vi "ThresholdAviMesure.vi"() -> ()   [LabVIEW 2015]
uses:
  <vilib>/vision/NI_Vision_Development_Module.lvlib
  <vilib>/ptbypt/NI_PtbyPt.lvlib
panel:
  out "Numero de Macthes 2":i32
  out "Dif. CM":dbl
  in  "x":i32=20
  out "Dif. Puntos":i32
  out "2°":i32
  out "1°":i32
  out "Global Rectangle":dbl[](array[numeric])
  in  "Tab Control":T1(tab)
  out "Waveform Chart":dbl(graph)
  out "Waveform Chart 2":dbl(graph)
  out "Waveform Chart 3":dbl(graph)
  out "Waveform Graph":dbl[](graph)
  out "Saving Data":bool
  in  "Filename":path=path "C:/Users/denni/Google Drive/ProyectoEspi/Dennis/Espirometro.lvm/Medidas.xlsx"
  out "Dist. CM":sgl
  out "Dist. Pixel":sgl
  out "Image 2":T2(plugin-control)
  out "Image":T2(plugin-control)
  out "Barra de Progreso":i32(slide) max=1548 scale=-1.0..1548.0
  out "SNAP 1":bool
  out "SNAP 2":bool
  out "Numero de Macthes":i32
  out "Coordenadas":T3(array[cluster]) {"Position"."Y" format="%.2f"; "Position"."X" format="%.2f"}
  in  "REC":bool=TRUE
  in  "SNAP 1":bool=TRUE
  in  "Stop Button":bool
  in  "Minimum Score":sgl=700.0
  in  "Max # of Matches":i32=1
  out "Threshold":T2(plugin-control)
  out "Original":T2(plugin-control)
  in  "Blue or Luminance":cluster{i32, i32}(slide)={30, 255} scale=0.0..255.0
  in  "Green or Saturation":cluster{i32, i32}(slide)={100, 255} scale=0.0..255.0
  in  "Threshold Color Mode":enum32{"RGB", "HSL"}(radio)=enum."HSL"
  in  "Red or Hue":cluster{i32, i32}(slide)={90, 222} scale=0.0..255.0
  out "error out":errorcluster
  in  "error in (no error)":errorcluster
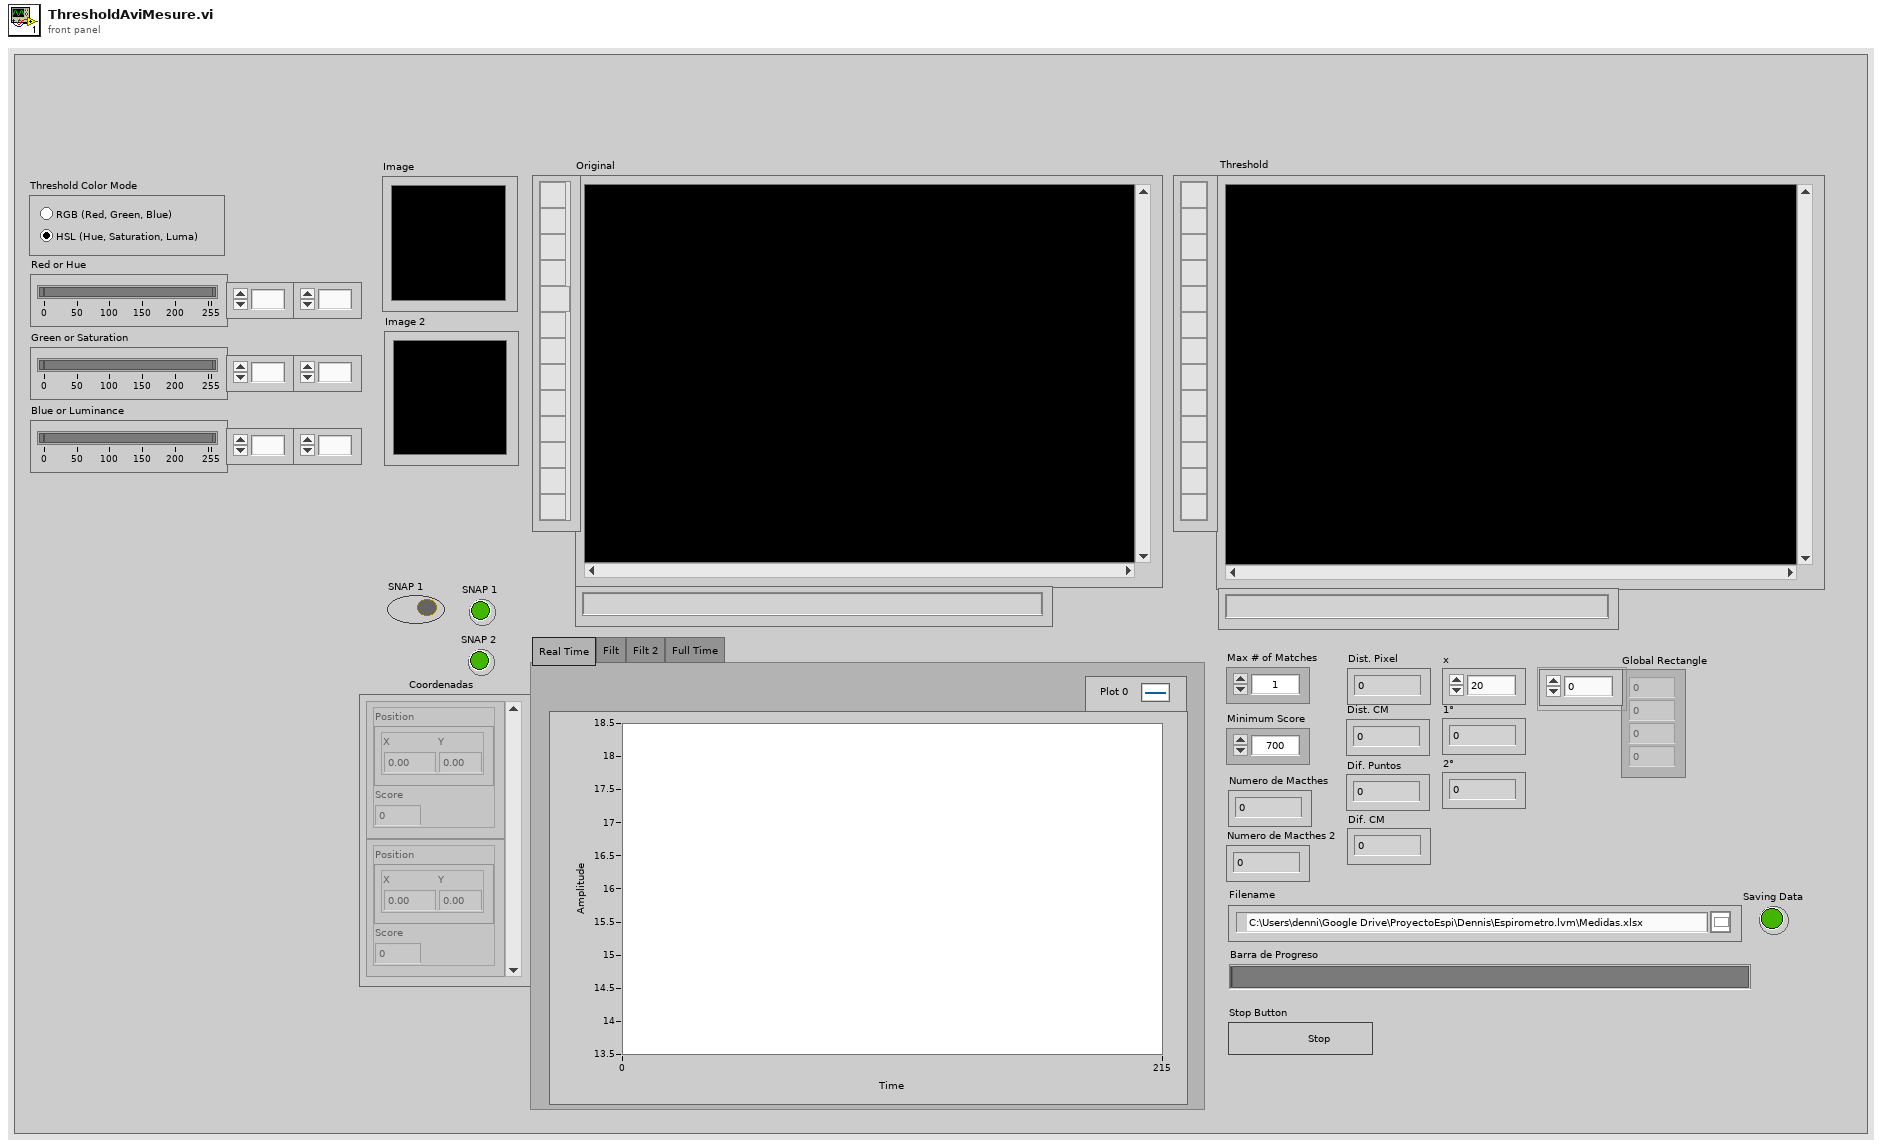
[diagram p1: front panel]
types:
  T1 = enum32{"Real Time", "Filt", "Filt 2", "Full Time"}
  T2 = typedef "IMAQ Image.ctl" = refnum<image>
  T3 = cluster{"Position":cluster{"X":dbl, "Y":dbl}, "Score":dbl}[]
  T4 = typedef "Image Type" = u32
  T5 = typedef "IMAQ AVI2 Refnum.ctl" = refnum<k20>
  T6 = cluster{"Global Rectangle":i32[], "Contours":cluster{"Contour Type":u32, "ROI Type":u32, "Points":i32[]}[]}
  T7 = cluster{"Position":cluster{"x":sgl, "y":sgl}, "Angle":sgl, "Scale":sgl, "Score":sgl, "Bounding Box":cluster{"x":sgl, "y":sgl}[]}[]
  T8 = cluster{"Position":cluster{"x":sgl, "y":sgl}, "Angle":sgl}
  T9 = cluster{"Position":cluster{"x":sgl, "y":sgl}, "Angle":sgl, "Scale":sgl, "Score":sgl, "Bounding Box":cluster{"x":sgl, "y":sgl}[]}
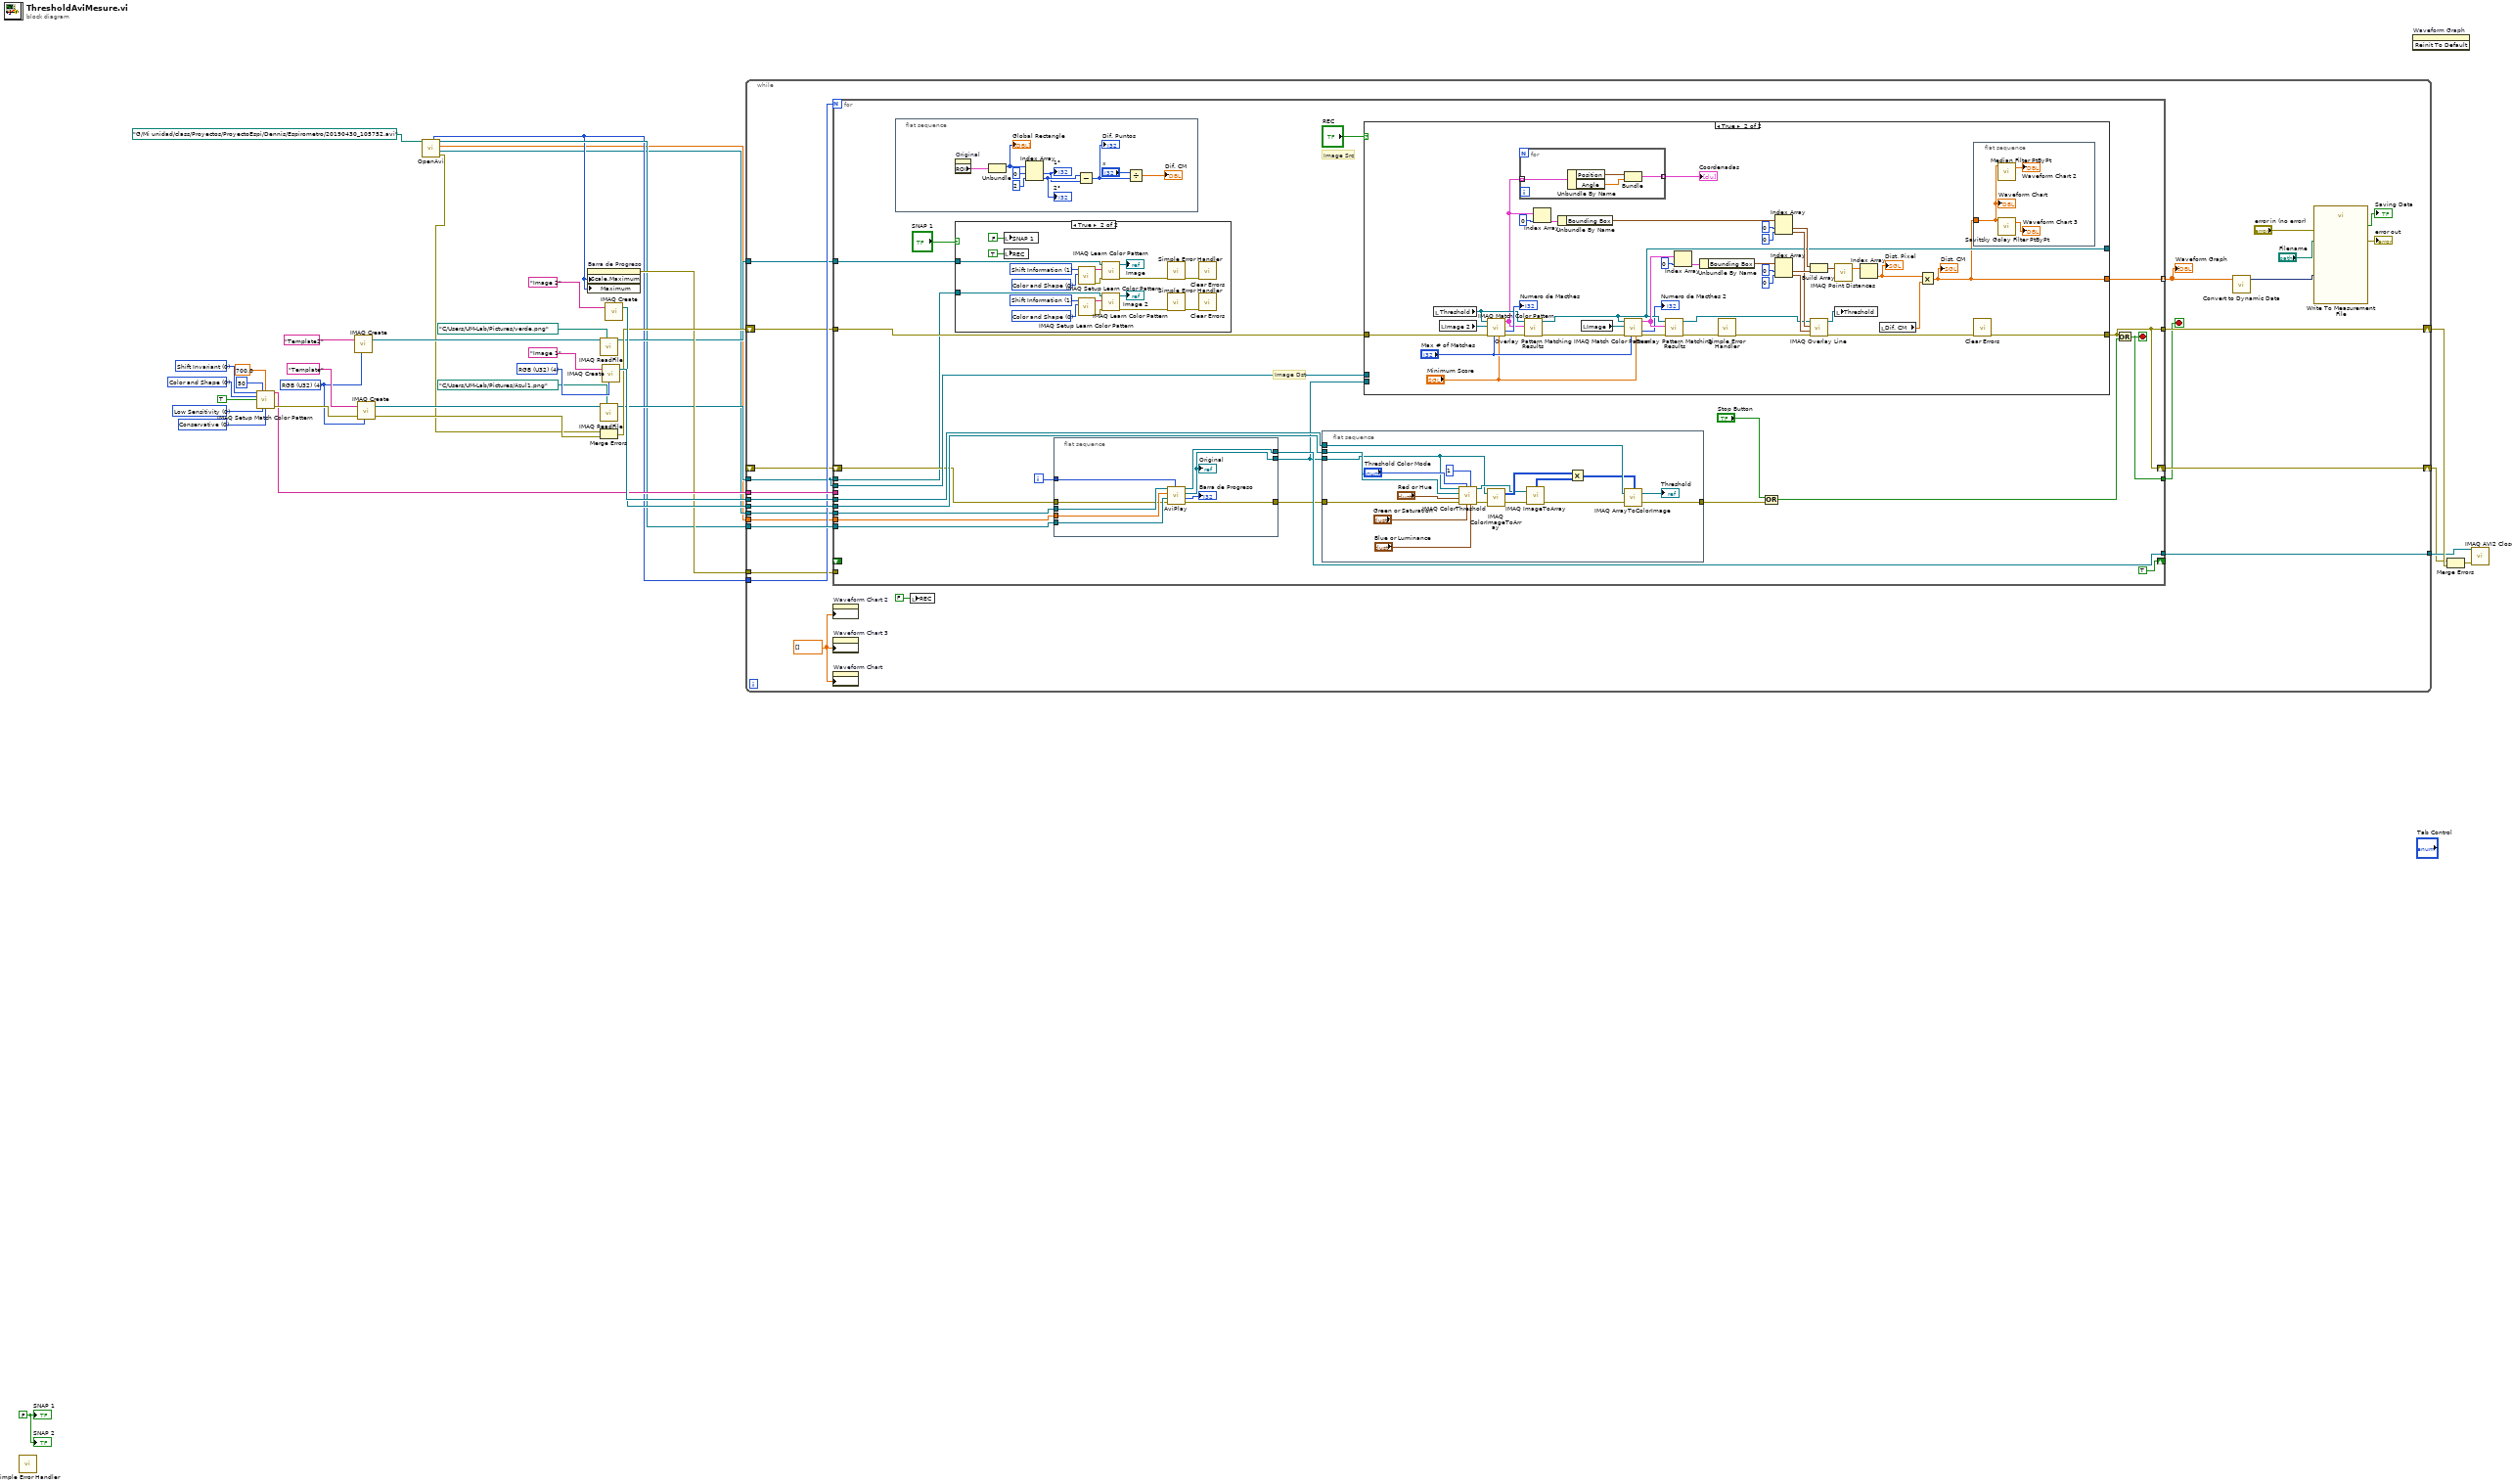
[diagram p0: block diagram]
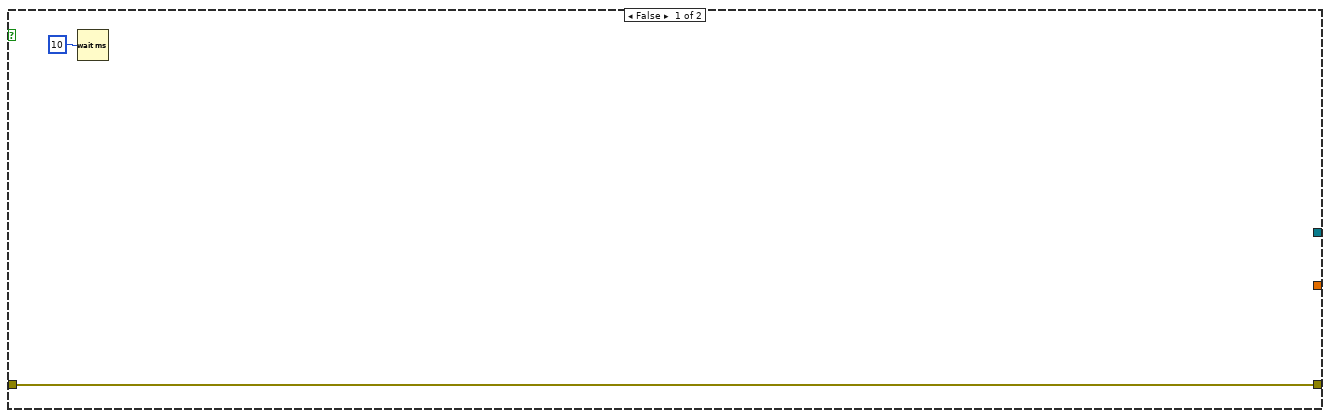
[diagram p3: hidden frame]
diagram:
  w17 = FALSE
  w24 = u32 0 items=["Shift Invariant", "Rotation Invariant"] ("Match Mode")
  w26 = u32 0 items=["Color and Shape", "Color", "Shape"] ("Match Feature Mode")
  w27 = u32 0 items=["Conservative", "Balance", "Aggressive", "Very Aggressive"] ("Search Strategy")
  w28 = u32 0 items=["Low Sensitivity", "Medium Sensitivity", "High Sensitivity"] ("Color Sensitivity")
  w18 = T4 4 items=["Grayscale (U8)", "Grayscale (I16)", "Grayscale (SGL)", "Complex (CSG)", "RGB (U32)", "HSL (U32)", "RGB (U64)", "Grayscale (U16)"] ("Image Type")
  w36 = T4 4 items=["Grayscale (U8)", "Grayscale (I16)", "Grayscale (SGL)", "Complex (CSG)", "RGB (U32)", "HSL (U32)", "RGB (U64)", "Grayscale (U16)"] ("Image Type")
  n1 = call <vilib>:"Simple Error Handler.vi"() -> ()  [unwired: 5 in, 5 out]
  n2 = call "IMAQ Setup Match Color Pattern"("Match Mode"=w24, "Minimum Contrast"=50, "Color Score Weight"=sgl 700.0, "Match Feature Mode"=w26, "Subpixel Accuracy"=TRUE, "Color Sensitivity"=w28, "Search Strategy"=w27) -> ("Match Color Pattern Setup Data"=w29:string, "error out"=w31:errorcluster)  [unwired: 7 in]
  n3 = call "IMAQ Create"("Image Name"="Template2", "Image Type"=w18) -> ("New Image"=w11:T2)  [unwired: 3 in, 1 out]
  n4 = call "IMAQ Create"("Image Name"="Template", "Image Type"=w18, "error in (no error)"=w31) -> ("New Image"=w13:T2, "error out"=w30:errorcluster)  [unwired: 2 in]
  n5 = call "OpenAvi.vi"("Example Image Path"=path "G:/Mi unidad/class/Proyectos/ProyectoEspi/Dennis/Espirometro/20190430_105752.avi" ("base path")) -> ("error out"=w5:errorcluster, "AVI Refnum (duplicate)"=w3:T5, "Sec per Frame"=w2:dbl, "Refnum out Image"=w6:T2, "Number of Frames For"=w4:u32)  [unwired: 6 in]
  n6 = property on="Barra de Progreso" class="Slide (strict)"("Scale.Maximum"=w4, "Maximum"=w4) -> (error out=w16:errorcluster)  [unwired: 2 in, 1 out]
  n7 = call "IMAQ ReadFile"("File Path"=path "C:/Users/UM-Lab/Pictures/verde.png", "Image"=w11) -> ("Image Out"=w10:T2)  [unwired: 5 in, 4 out]
  n8 = call "IMAQ ReadFile"("File Path"=path "C:/Users/UM-Lab/Pictures/Azul1.png", "Image"=w13) -> ("Image Out"=w12:T2)  [unwired: 5 in, 4 out]
  n9 = Merge Errors(w5, w30) -> (w21:errorcluster)
  n10 = call "IMAQ Create"("Image Name"="Image 1", "Image Type"=w36) -> ("New Image"=w35:T2)  [unwired: 3 in, 1 out]
  n11 = call "IMAQ Create"("Image Name"="Image 2") -> ("New Image"=w33:T2)  [unwired: 4 in, 1 out]
  n12 = while {
    tunnel: w35 -> [w61]
    tunnel: w33 -> [w60]
    tunnel: w29 -> [w59]
    tunnel: w12 -> [w42]
    tunnel: w10 -> [w41]
    tunnel: w6 -> [w56]
    tunnel: w4 -> [w55]
    tunnel: w16 -> [w54]
    tunnel: w2 -> [w53]
    tunnel: w3 -> [w52]
    shift-right: [w58] -> w20
    shift-left: w21 -> [w43]
    shift-right: [w57] -> w1
    shift-left: _ -> [w51]
    tunnel: [w50] -> w14
    stop <- w38 stop-if-true
    w39 = dbl[] [] ("History Data")
    n13 = for {
      N: w55 -> [_]
      tunnel: w56 -> [w78]
      shift-right: [w67] -> w57
      shift-left: w51 -> [w72]
      tunnel: w61 -> [w84]
      tunnel: w60 -> [w83]
      tunnel: w59 -> [_]
      tunnel: w43 -> [w81]
      tunnel: w42 -> [w80]
      shift-right: [TRUE] -> _
      shift-left: _ -> [_]
      tunnel: [w67] -> w58
      tunnel: w54 -> [_]
      tunnel: w53 -> [w75]
      tunnel: w52 -> [w77]
      tunnel: [w74] -> w50
      tunnel: [w79] -> w44 mode=indexing
      tunnel: w42 -> [w71]
      tunnel: w41 -> [w70]
      tunnel: [w62] -> w38
      i -> [w76]
      stop <- w62 stop-if-true
      # "Image Src"
      # "Image Dst"
      n14 = flat-sequence {
        frame #0 {
          n15 = property on="Original" class="ImageControl"() -> ("ROI"=w102:T6)  [unwired: 2 in, 2 out]
          n16 = Unbundle(w102) -> ("Global Rectangle"=w101:i32[])  [unwired: 1 out]
          "Global Rectangle" <- w101
          n17 = Index Array(array=w101, index #1=0 ("index"), index #2=2 ("index")) -> (element #1=w97:i32, element #2=w98:i32)
          "1°" <- w97
          "2°" <- w98
          n18 = Subtract(x=w98, y=w97) -> (x-y=w96:i32)
          "Dif. Puntos" <- w96
          n19 = Divide(x="x", y=w96) -> (x/y=→"Dif. CM":dbl)
        }
      }
      n20 = case shown="True" "SNAP 1" {
        tunnel: w70 -> [_ w123]
        tunnel: w71 -> [_ w122]
        frame False {
        }
        frame True {
          w127 = u32 0 items=["Color and Shape", "Color", "Shape "] ("Feature Mode")
          w128 = u32 1 items=["All", "Shift Information", "Rotation Information"] ("Learn Mode")
          w138 = u32 0 items=["Color and Shape", "Color", "Shape "] ("Feature Mode")
          w137 = u32 1 items=["All", "Shift Information", "Rotation Information"] ("Learn Mode")
          n21 = local write "SNAP 1"(FALSE ("Boolean")) -> ()
          n22 = local write "REC"(TRUE ("REC")) -> ()
          n23 = call "IMAQ Setup Learn Color Pattern"("Feature Mode"=w138, "Learn Mode"=w137) -> ("error out"=w135:errorcluster, "Learn Color Pattern Setup Data"=w136:string)  [unwired: 8 in]
          n24 = call "IMAQ Setup Learn Color Pattern"("Feature Mode"=w127, "Learn Mode"=w128) -> ("error out"=w125:errorcluster, "Learn Color Pattern Setup Data"=w124:string)  [unwired: 8 in]
          n25 = call "IMAQ Learn Color Pattern"("error in (no error)"=w135, "Learn Color Pattern Setup Data"=w136, "Image"=w123) -> ("error out"=w133:errorcluster, "Template Image Out"=→"Image":T2)  [unwired: 7 in]
          n26 = call "IMAQ Learn Color Pattern"("error in (no error)"=w125, "Learn Color Pattern Setup Data"=w124, "Image"=w122) -> ("error out"=w129:errorcluster, "Template Image Out"=→"Image 2":T2)  [unwired: 7 in]
          n27 = call <vilib>:"Simple Error Handler.vi"("error in (no error)"=w133) -> ("error out"=w132:errorcluster)  [unwired: 4 in, 4 out]
          n28 = call <vilib>:"Simple Error Handler.vi"("error in (no error)"=w129) -> ("error out"=w126:errorcluster)  [unwired: 4 in, 4 out]
          n29 = call <vilib>:"Clear Errors.vi"("error in (no error)"=w132) -> ()  [unwired: 5 in, 2 out]
          n30 = call <vilib>:"Clear Errors.vi"("error in (no error)"=w126) -> ()  [unwired: 5 in, 2 out]
        }
      }
      n31 = flat-sequence {
        tunnel: w78 -> [w93]
        tunnel: w77 -> [w92]
        tunnel: w76 -> [w91]
        tunnel: w75 -> [w90]
        tunnel: [w89] -> w74
        tunnel: [w87] -> w73
        tunnel: w72 -> [w86]
        tunnel: [w85] -> w66
        frame #0 {
          n32 = call "AviPlay.vi"("Numeric Iteration"=w91, "error in (no error)"=w86, "New Image"=w93, "Seconds per Frame"=w90, "Refnum in Avi"=w92) -> ("error out"=w85:errorcluster, "Progress Bar"=→"Barra de Progreso":i32, "Image Out"=w87:T2, "Refnum out Avi"=w89:T5)  [unwired: 3 in]
          "Original" <- w87
        }
      }
      n33 = flat-sequence {
        tunnel: w84 -> [w115]
        tunnel: w83 -> [w111]
        tunnel: w73 -> [w108]
        tunnel: w66 -> [w107]
        tunnel: [w103] -> w63
        frame #0 {
          n34 = call "IMAQ ColorThreshold"("Blue or Luma or Val or Inten Range"="Blue or Luminance", "Replace Value"=1, "Green or Sat Range"="Green or Saturation", "Color Mode"="Threshold Color Mode", "error in (no error)"=w107, "Red or Hue Range"="Red or Hue", "Image Dst"=w111, "Image Src"=w108) -> ("error out"=w106:errorcluster, "Image Dst Out"=w116:T2)  [unwired: 2 in]
          n35 = call "IMAQ ColorImageToArray"("Image"=w108, "error in (no error)"=w106) -> ("Image Pixels (U32)"=w117:u32[][], "error out"=w105:errorcluster)  [unwired: 2 in, 1 out]
          n36 = call "IMAQ ImageToArray"("error in (no error)"=w105, "Image"=w116) -> ("error out"=w104:errorcluster, "Image Pixels (U8)"=w112:u8[][])  [unwired: 2 in, 3 out]
          n37 = Multiply(x=w117, y=w112) -> (x*y=w114:u32[][])
          n38 = call "IMAQ ArrayToColorImage"("Image Pixels (U32)"=w114, "Image"=w115, "error in (no error)"=w104) -> ("Image Out"=→"Threshold":T2, "error out"=w103:errorcluster)  [unwired: 2 in]
        }
      }
      n39 = case shown="True" "REC" {
        tunnel: [_ w156] -> _
        tunnel: [w139 w177] -> w67
        tunnel: w73 -> [_ _]
        tunnel: w80 -> [_ _]
        tunnel: w81 -> [w139 w147]
        tunnel: [_ w141] -> w79
        frame False {
          n40 = Wait (ms)(milliseconds to wait=u32 10) -> ()  [unwired: 1 out]
        }
        frame True {
          n41 = local read "Threshold"() -> (w176:T2)
          n42 = local read "Image 2"() -> (w175:T2)
          n43 = call "IMAQ Match Color Pattern"("Minimum Match Score"="Minimum Score", "Number of Matches Requested"="Max # of Matches", "error in (no error)"=w147, "Template Image"=w175, "Image"=w176) -> ("error out"=w178:errorcluster, "Number of Matches"=→"Numero de Macthes":i32, "Matches"=w170:T7)  [unwired: 4 in]
          n44 = for {
            tunnel: w170 -> [w187] mode=indexing
            tunnel: [w184] -> w179 mode=indexing
            n45 = Unbundle By Name(w187) -> ("Position"=w186:cluster{"x":sgl, "y":sgl}, "Angle"=w185:sgl)
            n46 = Bundle("Position"=w186, "Angle"=w185) -> (w184:T8)  [unwired: 1 in]
          }
          "Coordenadas" <- w179
          n47 = call "Overlay Pattern Matching Results.vi"("error in"=w178, "Matches"=w170, "Image"=w176) -> ("error out"=w146:errorcluster, "Image Out"=w156:T2)  [unwired: 7 in]
          n48 = Index Array(array=w170, index=0) -> (element=w167:T9)
          n49 = Unbundle By Name(w167) -> ("Bounding Box"=w166:cluster{"x":sgl, "y":sgl}[])
          n50 = local read "Image"() -> (w174:T2)
          n51 = call "IMAQ Match Color Pattern"("Minimum Match Score"="Minimum Score", "Number of Matches Requested"="Max # of Matches", "error in (no error)"=w146, "Template Image"=w174, "Image"=w156) -> ("error out"=w173:errorcluster, "Number of Matches"=→"Numero de Macthes 2":i32, "Matches"=w169:T7)  [unwired: 4 in]
          n52 = call "Overlay Pattern Matching Results.vi"("error in"=w173, "Matches"=w169, "Image"=w156) -> ("error out"=w172:errorcluster, "Image Out"=w145:T2)  [unwired: 7 in]
          n53 = Index Array(array=w169, index=0) -> (element=w163:T9)
          n54 = Unbundle By Name(w163) -> ("Bounding Box"=w162:cluster{"x":sgl, "y":sgl}[])
          n55 = call <vilib>:"Simple Error Handler.vi"("error in (no error)"=w172) -> ("error out"=w143:errorcluster)  [unwired: 4 in, 4 out]
          n56 = Index Array(array=w166, index #1=0 ("index"), index #2=0 ("index")) -> (element #1=w159:cluster{"x":sgl, "y":sgl}, element #2=w157:cluster{"x":sgl, "y":sgl})
          n57 = Index Array(array=w162, index #1=0 ("index"), index #2=0 ("index")) -> (element #1=w160:cluster{"x":sgl, "y":sgl}, element #2=w152:cluster{"x":sgl, "y":sgl})
          n58 = Build Array(w159, w160) -> (w164:cluster{"x":sgl, "y":sgl}[])
          n59 = call "IMAQ Overlay Line"("error in (no error)"=w143, "End Point"=w152, "Start Point"=w157, "Image"=w145) -> ("error out"=w142:errorcluster, "Image Out"=w153:T2)  [unwired: 6 in]
          n60 = call "IMAQ Point Distances"("Points"=w164) -> ("Distances"=w154:sgl[])  [unwired: 4 in, 1 out]
          n61 = local write "Threshold"(w153) -> ()
          n62 = Index Array(array=w154) -> (element=w151:sgl)  [unwired: 1 in]
          "Dist. Pixel" <- w151
          n63 = local read "Dif. CM"() -> (w150:dbl)
          n64 = Multiply(x=w151, y=w150) -> (x*y=w141:dbl)
          "Dist. CM" <- w141
          n65 = flat-sequence {
            tunnel: w141 -> [w182]
            frame #0 {
              n66 = call <vilib>:"Median Filter PtByPt.vi"("x"=w182) -> ("Filtered x"=→"Waveform Chart 2":dbl)  [unwired: 3 in, 1 out]
              n67 = call <vilib>:"Savitzky Golay Filter PtByPt.vi"("x"=w182) -> ("Filtered x"=→"Waveform Chart 3":dbl)  [unwired: 3 in, 1 out]
              "Waveform Chart" <- w182
            }
          }
          n68 = call <vilib>:"Clear Errors.vi"("error in (no error)"=w142) -> ("error out"=w177:errorcluster)  [unwired: 5 in, 1 out]
        }
      }
      n69 = Or(x="Stop Button", y=w63) -> (x .or. y?=w64:bool)
      n70 = Or(x=w67, y=w64) -> (x .or. y?=w62:bool)
    }
    "Waveform Graph" <- w44
    n71 = property on="Waveform Chart 2" class="WFChart (strict)"("History Data"=w39) -> ()  [unwired: 2 in, 2 out]
    n72 = property on="Waveform Chart 3" class="WFChart (strict)"("History Data"=w39) -> ()  [unwired: 2 in, 2 out]
    n73 = property on="Waveform Chart" class="WFChart (strict)"("History Data"=w39) -> ()  [unwired: 2 in, 2 out]
    n74 = local write "REC"(FALSE ("REC")) -> ()
    n75 = call "Convert to Dynamic Data"("Array"=w44) -> ("Dynamic Data Type"=w47:dynamicdata)  [unwired: 3 in]
    n76 = call "Write To Measurement File"("Signals"=w47, "error in (no error)"="error in (no error)", "Filename"="Filename") -> ("Saving Data"=→"Saving Data":bool, "error out"=→"error out":errorcluster)  [unwired: 14 in, 1 out]
  }
  n77 = invoke on="Waveform Graph" class="WFGraph (strict)" method="Reinit To Default"() -> ()  [unwired: 3 in, 3 out]
  n78 = Merge Errors(w1, w20) -> (w15:errorcluster)
  n79 = call "IMAQ AVI2 Close"("error in (no error)"=w15, "AVI Refnum"=w14) -> ()  [unwired: 10 out]
  "SNAP 2" <- w17
  "SNAP 1" <- w17
